vi "Run_6_of_6_Tests.vi"() -> ()   [LabVIEW 2019]
uses:
  <vilib>/Rock Robotics/WPI/ThirdParty/JAS_Junk/TrajLib/Trajectory_Library.lvlib
panel:
  out "Lead Lag":bool
  out "Pose3d":bool
  out "Transform3d":bool
  out "Rotation3d":bool
  out "Translation3d":bool
  out "Twist3d":bool
  out "Function Generator \nMatrix":bool
  out "LTV Unicycle \nController":bool
  out "LTV Diff Drive \nController":bool
  out "Time Interpolatable Rotation":bool
  out "Time Interpolatable Double":bool
  out "Time Interpolatable Boolean":bool
  out "Time Interpolatable Pose":bool
  out "Implicit Model Follower":bool
  out "Function Generator":bool
  out "Diff Drive Accel Limiter":bool
  out "String":string
  out "All Tests Finished":bool
  # "FORMAL TRAJECTORY / CONTROL LIBRARY TEST PROCEDURE"
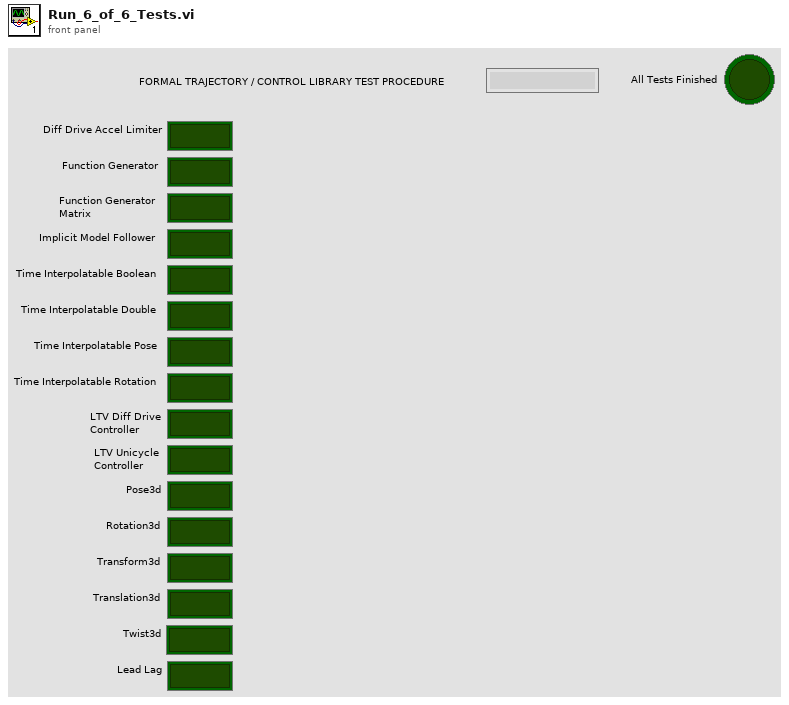
[diagram p1: front panel]
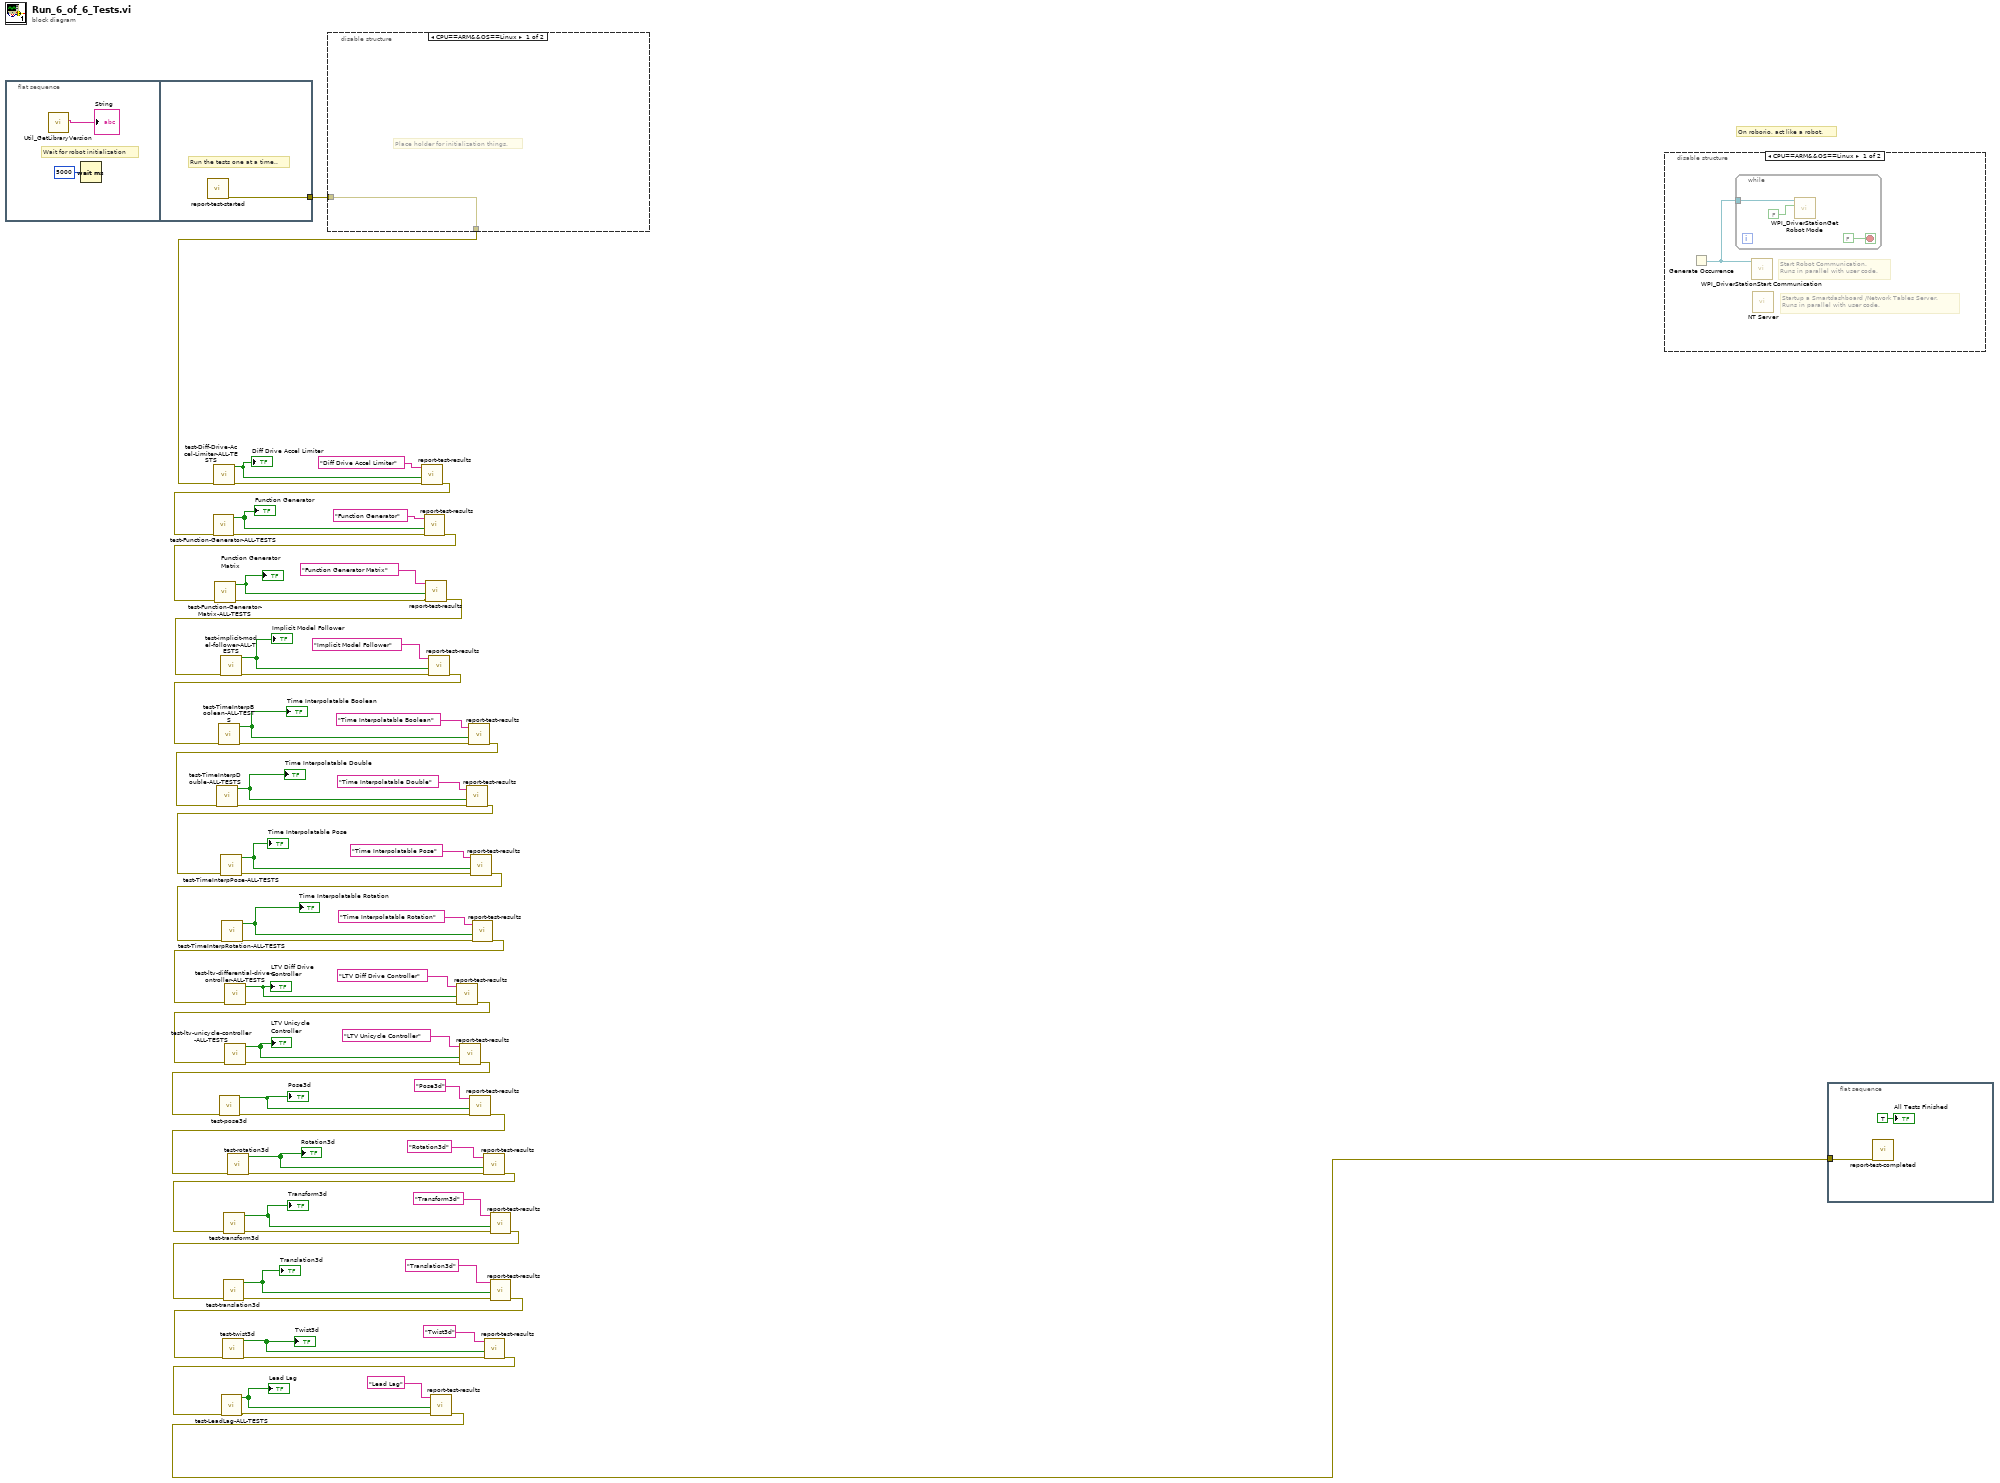
[diagram p0: block diagram]
diagram:
  # "On roborio, act like a robot."
  n1 = flat-sequence {
    tunnel: [w69] -> w66
    frame #0 {
      # "Wait for robot initialization"
      n2 = call <vilib>:"Util_GetLibraryVersion.vi"() -> ("TrajLibVersion"=→"String":string)  [unwired: 11 in]
      n3 = Wait (ms)(milliseconds to wait=u32 5000) -> ()  [unwired: 1 out]
    }
    frame #1 {
      # "Run the tests one at a time.."
      n4 = call "report-test-started.vi"() -> ("error out"=w69:errorcluster)  [unwired: 11 in]
    }
  }
  n5 = disable-structure shown="CPU==ARM&&OS==Linux" {
    disable-tunnel: w66 -> [w70 w71]
    disable-tunnel: [w70 w71] -> w62
    frame condition #0 {
      # "Place holder for initialization things."
    }
    frame condition #1 (active) {
    }
  }
  n6 = call "test-Diff-Drive-Accel-Limiter-ALL-TESTS.vi"("error in (no error)"=w62) -> ("error out"=w64:errorcluster, "All Passed"=w63:bool)  [unwired: 9 in]
  "Diff Drive Accel Limiter" <- w63
  n7 = call "report-test-results.vi"("error in (no error)"=w64, "TestPassed"=w63, "Test Name"="Diff Drive Accel Limiter") -> ("error out"=w58:errorcluster)  [unwired: 8 in]
  n8 = call "test-Function-Generator-ALL-TESTS.vi"("error in (no error)"=w58) -> ("error out"=w60:errorcluster, "All Passed"=w59:bool)  [unwired: 9 in]
  "Function Generator" <- w59
  n9 = call "report-test-results.vi"("error in (no error)"=w60, "TestPassed"=w59, "Test Name"="Function Generator") -> ("error out"=w28:errorcluster)  [unwired: 8 in]
  n10 = call "test-Function-Generator-Matrix-ALL-TESTS.vi"("error in (no error)"=w28) -> ("error out"=w30:errorcluster, "All Passed"=w29:bool)  [unwired: 9 in]
  "Function Generator \nMatrix" <- w29
  n11 = call "report-test-results.vi"("error in (no error)"=w30, "TestPassed"=w29, "Test Name"="Function Generator Matrix") -> ("error out"=w27:errorcluster)  [unwired: 8 in]
  n12 = call "test-implicit-model-follower-ALL-TESTS.vi"("error in (no error)"=w27) -> ("error out"=w56:errorcluster, "All Passed"=w55:bool)  [unwired: 9 in]
  "Implicit Model Follower" <- w55
  n13 = call "report-test-results.vi"("error in (no error)"=w56, "TestPassed"=w55, "Test Name"="Implicit Model Follower") -> ("error out"=w42:errorcluster)  [unwired: 8 in]
  n14 = call "test-TimeInterpBoolean-ALL-TESTS.vi"("error in (no error)"=w42) -> ("error out"=w50:errorcluster, "All Passed"=w47:bool)  [unwired: 9 in]
  "Time Interpolatable Boolean" <- w47
  n15 = call "report-test-results.vi"("error in (no error)"=w50, "TestPassed"=w47, "Test Name"="Time Interpolatable Boolean") -> ("error out"=w39:errorcluster)  [unwired: 8 in]
  n16 = call "test-TimeInterpDouble-ALL-TESTS.vi"("error in (no error)"=w39) -> ("error out"=w48:errorcluster, "All Passed"=w46:bool)  [unwired: 9 in]
  "Time Interpolatable Double" <- w46
  n17 = call "report-test-results.vi"("error in (no error)"=w48, "TestPassed"=w46, "Test Name"="Time Interpolatable Double") -> ("error out"=w40:errorcluster)  [unwired: 8 in]
  n18 = call "test-TimeInterpPose-ALL-TESTS.vi"("error in (no error)"=w40) -> ("error out"=w53:errorcluster, "All Passed"=w52:bool)  [unwired: 9 in]
  "Time Interpolatable Pose" <- w52
  n19 = call "report-test-results.vi"("error in (no error)"=w53, "TestPassed"=w52, "Test Name"="Time Interpolatable Pose") -> ("error out"=w41:errorcluster)  [unwired: 8 in]
  n20 = call "test-TimeInterpRotation-ALL-TESTS.vi"("error in (no error)"=w41) -> ("error out"=w44:errorcluster, "All Passed"=w43:bool)  [unwired: 9 in]
  "Time Interpolatable Rotation" <- w43
  n21 = call "report-test-results.vi"("error in (no error)"=w44, "TestPassed"=w43, "Test Name"="Time Interpolatable Rotation") -> ("error out"=w32:errorcluster)  [unwired: 8 in]
  n22 = call "test-ltv-differential-drive-controller-ALL-TESTS.vi"("error in (no error)"=w32) -> ("error out"=w35:errorcluster, "All Passed"=w36:bool)  [unwired: 9 in]
  "LTV Diff Drive \nController" <- w36
  n23 = call "report-test-results.vi"("error in (no error)"=w35, "TestPassed"=w36, "Test Name"="LTV Diff Drive Controller") -> ("error out"=w14:errorcluster)  [unwired: 8 in]
  n24 = call "test-ltv-unicycle-controller-ALL-TESTS.vi"("error in (no error)"=w14) -> ("error out"=w34:errorcluster, "All Passed"=w33:bool)  [unwired: 9 in]
  "LTV Unicycle \nController" <- w33
  n25 = call "report-test-results.vi"("error in (no error)"=w34, "TestPassed"=w33, "Test Name"="LTV Unicycle Controller") -> ("error out"=w7:errorcluster)  [unwired: 8 in]
  n26 = call "test-pose3d.vi"("error in (no error)"=w7) -> ("error out"=w9:errorcluster, "All PASSED"=w8:bool)  [unwired: 9 in]
  "Pose3d" <- w8
  n27 = call "report-test-results.vi"("error in (no error)"=w9, "TestPassed"=w8, "Test Name"="Pose3d") -> ("error out"=w6:errorcluster)  [unwired: 8 in]
  n28 = call "test-rotation3d.vi"("error in (no error)"=w6) -> ("error out"=w19:errorcluster, "ALL TESTS PASSED"=w18:bool)  [unwired: 9 in]
  "Rotation3d" <- w18
  n29 = call "report-test-results.vi"("error in (no error)"=w19, "TestPassed"=w18, "Test Name"="Rotation3d") -> ("error out"=w13:errorcluster)  [unwired: 8 in]
  n30 = call "test-transform3d.vi"("error in (no error)"=w13) -> ("error out"=w16:errorcluster, "All PASSED"=w15:bool)  [unwired: 9 in]
  "Transform3d" <- w15
  n31 = call "report-test-results.vi"("error in (no error)"=w16, "TestPassed"=w15, "Test Name"="Transform3d") -> ("error out"=w12:errorcluster)  [unwired: 8 in]
  n32 = call "test-translation3d.vi"("error in (no error)"=w12) -> ("error out"=w22:errorcluster, "All PASSED"=w21:bool)  [unwired: 9 in]
  "Translation3d" <- w21
  n33 = call "report-test-results.vi"("error in (no error)"=w22, "TestPassed"=w21, "Test Name"="Translation3d") -> ("error out"=w11:errorcluster)  [unwired: 8 in]
  n34 = call "test-twist3d.vi"("error in (no error)"=w11) -> ("error out"=w25:errorcluster, "All PASSED"=w24:bool)  [unwired: 9 in]
  "Twist3d" <- w24
  n35 = call "report-test-results.vi"("error in (no error)"=w25, "TestPassed"=w24, "Test Name"="Twist3d") -> ("error out"=w2:errorcluster)  [unwired: 8 in]
  n36 = call "test-LeadLag-ALL-TESTS.vi"("error in (no error)"=w2) -> ("error out"=w4:errorcluster, "All Passed"=w3:bool)  [unwired: 9 in]
  "Lead Lag" <- w3
  n37 = call "report-test-results.vi"("error in (no error)"=w4, "TestPassed"=w3, "Test Name"="Lead Lag") -> ("error out"=w1:errorcluster)  [unwired: 8 in]
  n38 = disable-structure shown="CPU==ARM&&OS==Linux" {
    frame condition #0 {
      # "Startup a Smartdashboard /Network Tables Server.\nRuns in parallel with user code."
      # "Start Robot Communication.\nRuns in parallel with user code."
      n39 = Generate Occurrence() -> (w72:refnum<k4>)
      n40 = while {
        tunnel: w72 -> [w75]
        stop <- FALSE stop-if-true
        n41 = call <vilib>:"WPI_DriverStationGet Robot Mode.vi"("Finish"=FALSE, "DS Occurrence"=w75) -> ()  [unwired: 10 out]
      }
      n42 = call <vilib>:"WPI_DriverStationStart Communication.vi"("occurrence"=w72) -> ()  [unwired: 2 in, 9 out]
      n43 = call <vilib>:"NT Server.vi"() -> ()  [unwired: 12 in]
    }
    frame condition #1 (active) {
    }
  }
  n44 = flat-sequence {
    tunnel: w1 -> [w76]
    frame #0 {
      n45 = call "report-test-completed.vi"("error in (no error)"=w76) -> ()  [unwired: 10 in, 1 out]
      "All Tests Finished" <- TRUE ("All Tests Finished")
    }
  }
